vi "UI Chip Fitting.vi"(8 "error in":errorcluster) -> (0 "error out":errorcluster)   [LabVIEW 2019, in "Test.lvlib"]
uses:
  Test.lvlib
  Fluidic Process/SubVI/Fluidic Para.ctl
  <vilib>/Utility/file.llb/Read Delimited Spreadsheet (string).vi
  Controller/Controller.lvlib
  Queues/Queues.lvlib
  Fluidic Process/Fluidic Process.lvlib
  IO/sbRIO9623/sbRIO9623.lvlib
  Selection Valve/IDEX/IDEX.lvlib
panel:
  out "SW 2":bool
  out "SW 1":bool
  out "FW 2":bool
  out "FW 1":bool
  out "REA":bool
  out "V1":bool
  out "V2":bool
  out "BR1":bool
  out "BR2":bool
  out "BL1":bool
  out "BL2":bool
  in  "Air Tight":bool
  in  "Purge":bool
  in  "Flow Rate":bool
  in  "Chip Hold Pressure":bool
  in  "SW1/2":bool
  in  "FW1/2":bool
  in  "REA":bool
  in  "V1+BR1":bool
  in  "V2+BR2":bool
  in  "BR1":bool
  in  "BR2":bool
  in  "BL1":bool
  in  "BL2":bool
  in  "Stop Process":bool
  out "Remaining Time(s)":dbl
  out "Total Process":string
  out "Current Process":string
  out "Gauge":dbl(knob)=1.2869315802184793e-48 scale=0.0..100.0
  in  "Buffer Load R":bool
  in  "Buffer Load L":bool
  in  "Back":bool
  # "/"
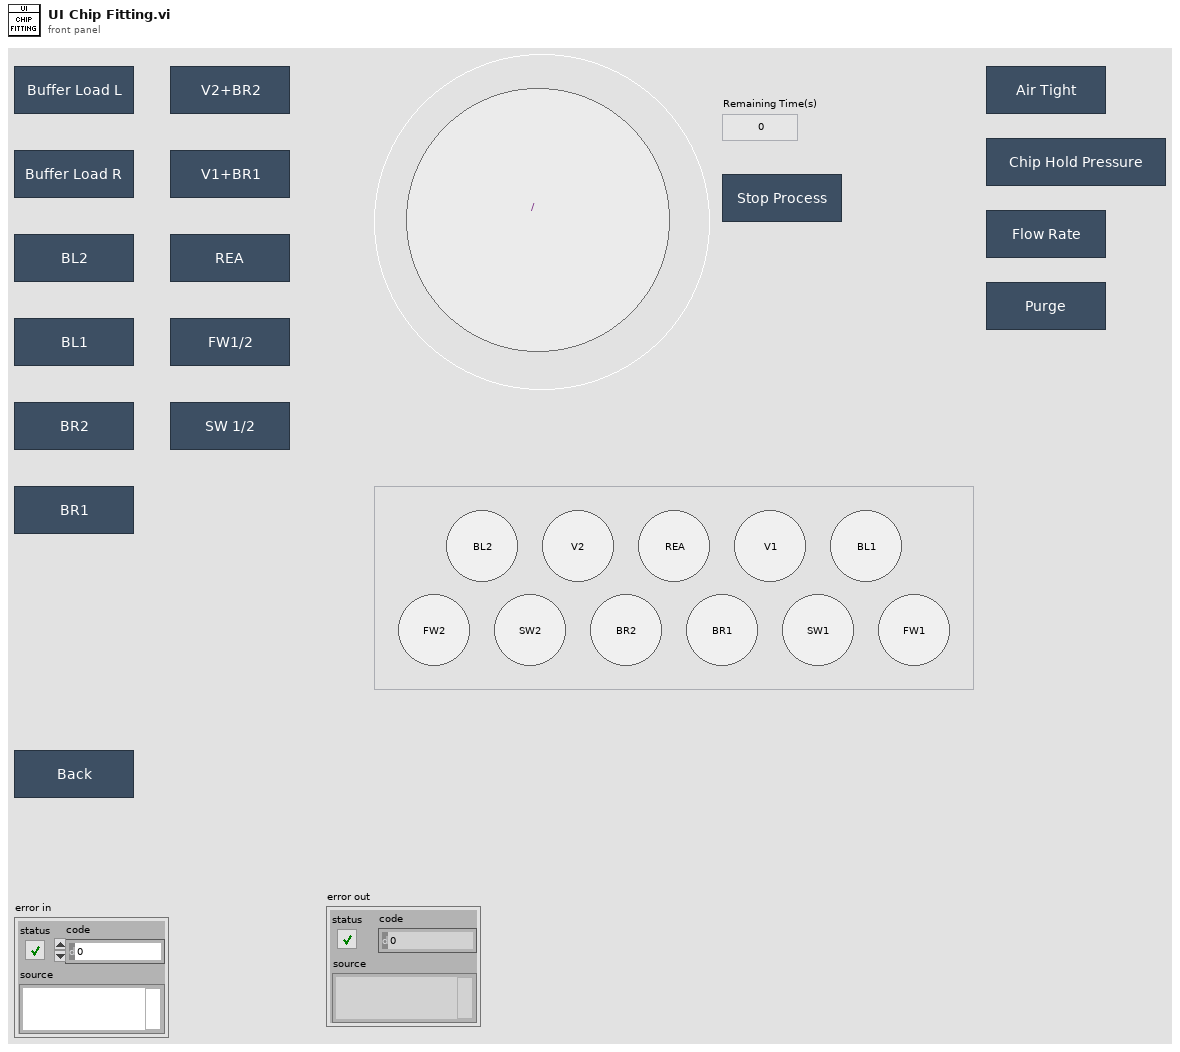
[diagram p1: front panel]
types:
  T1 = enum8{"Enabled", "Disabled", "Disabled and Grayed Out"}
  T2 = typedef "Fluidic Process.lvlib/Fluidic Para.ctl" = cluster{"Read Force Sensor":i32, "Read Regulator":i32, "Read Force Sensor?":bool, "Read Regulator?":bool, "Read Syringe Pump":i32, "Read Syringe Pump?":bool}
  T3 = enum16{"No Action", "Position 1", "Position 2", "Position 3", "Position 4", "Position 5", "Position 6"}
  T4 = typedef "Fluidic Process.lvlib/SEQ Data.ctl" = cluster{"Fluidic Process Done?":bool, "Current Process":i32, "Remaining Time":dbl, "Total Process":i32, "Air Sealing":bool, "Force Condition":bool}
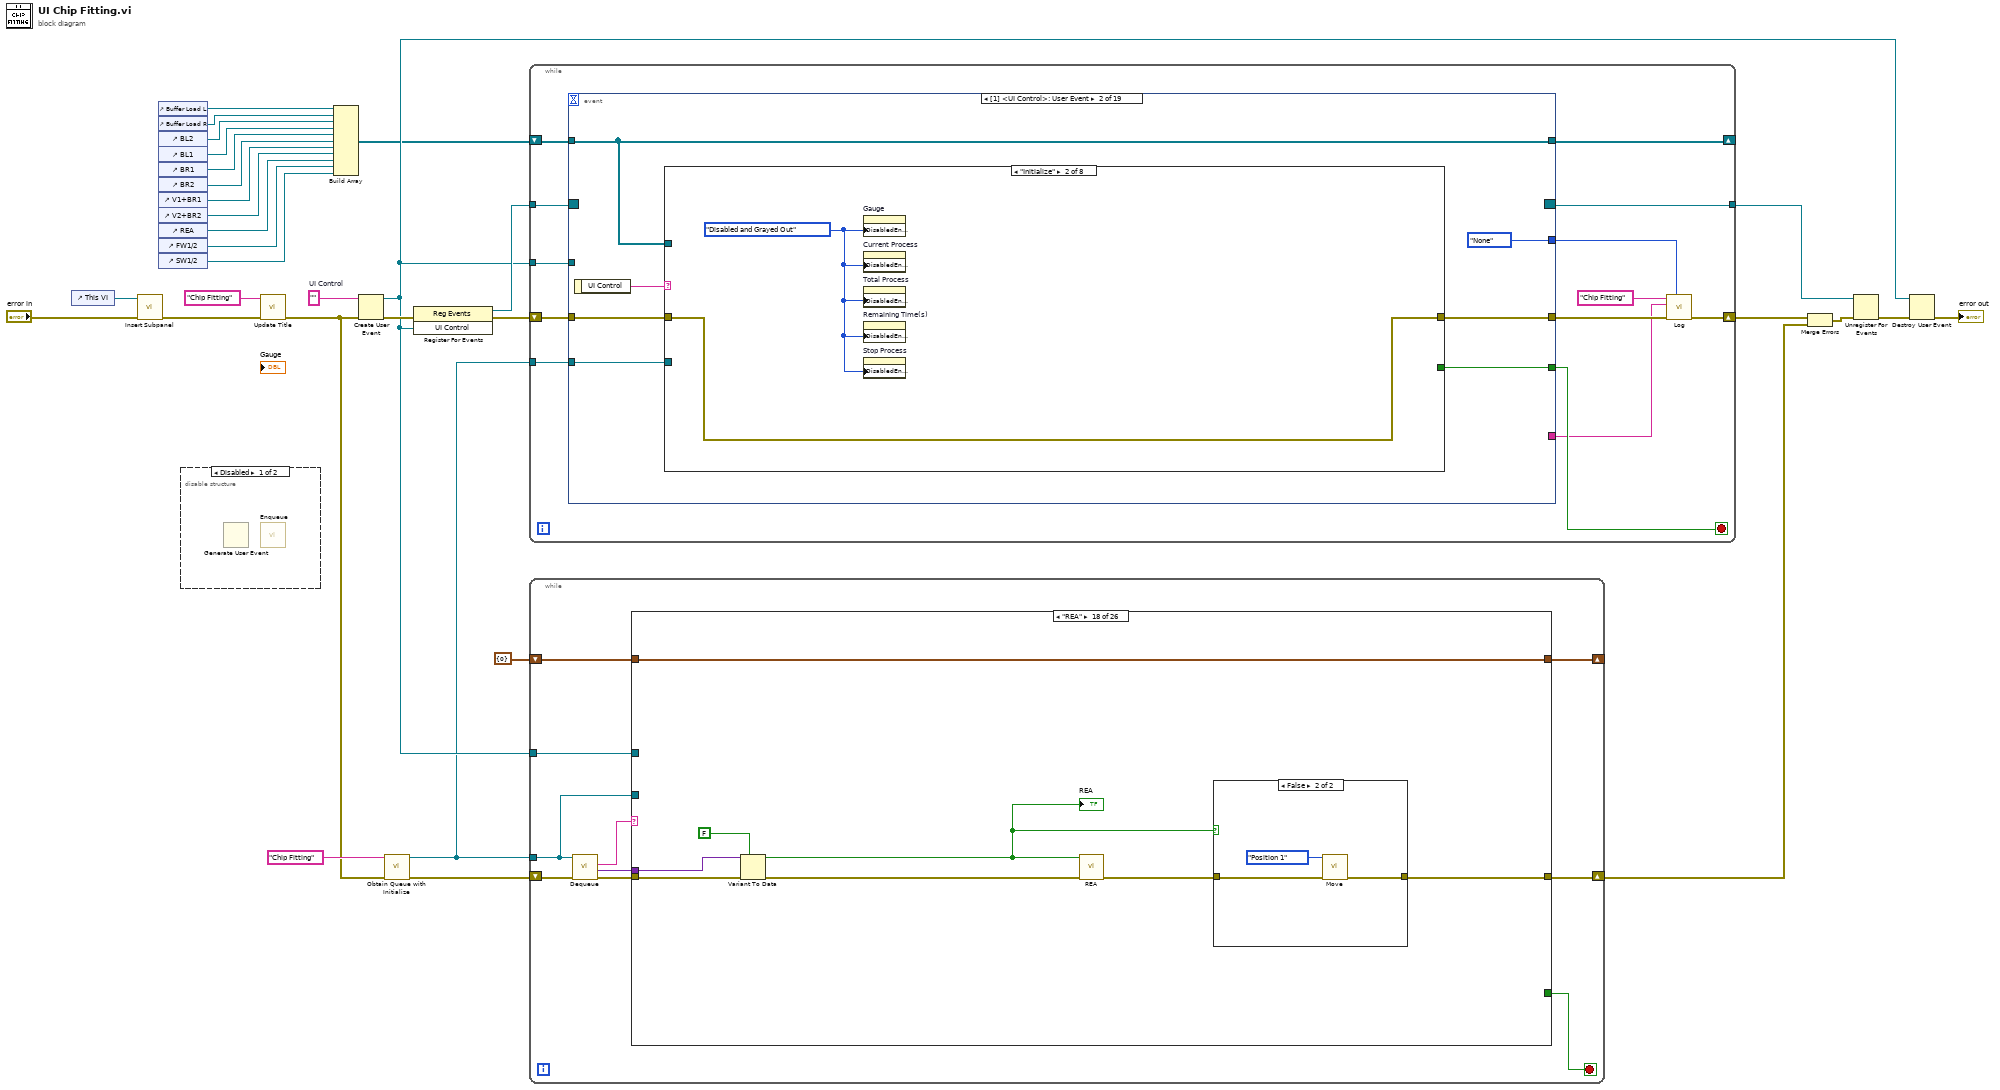
[diagram p0: block diagram]
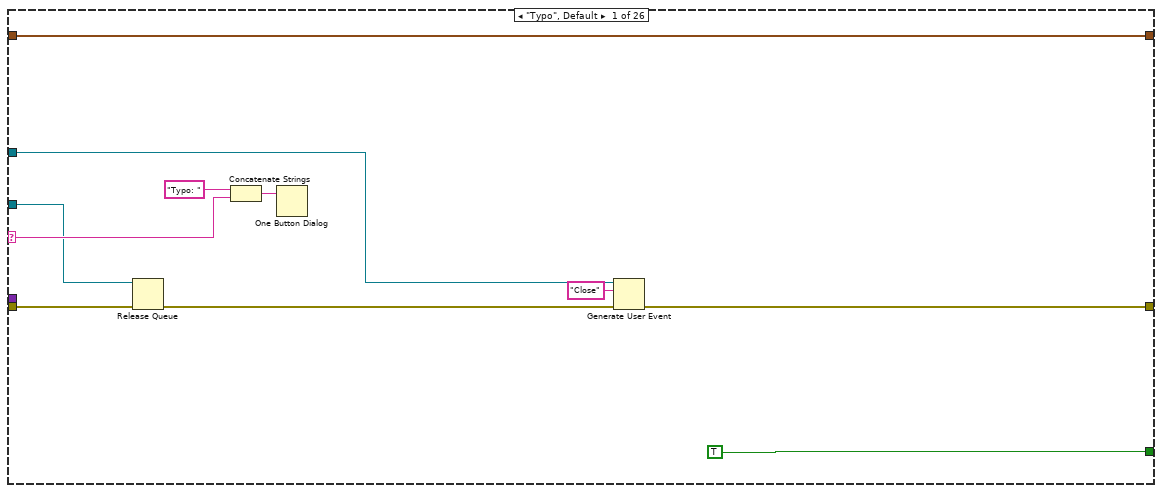
[diagram p3: hidden frame]
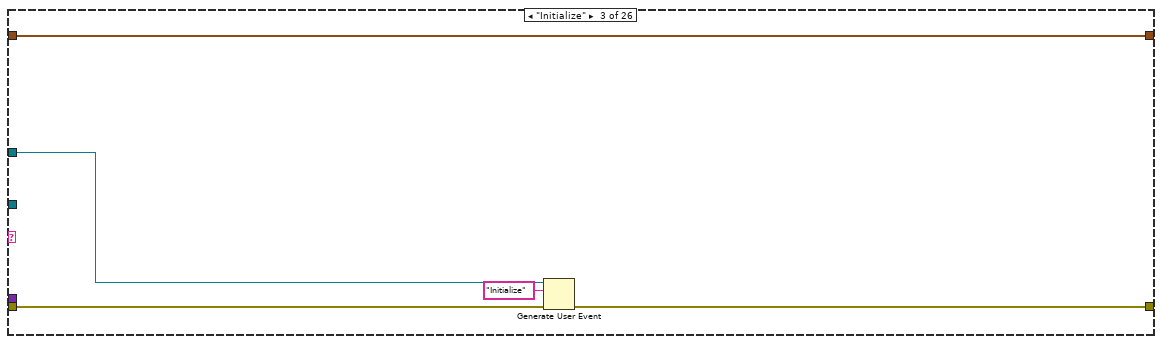
[diagram p5: hidden frame]
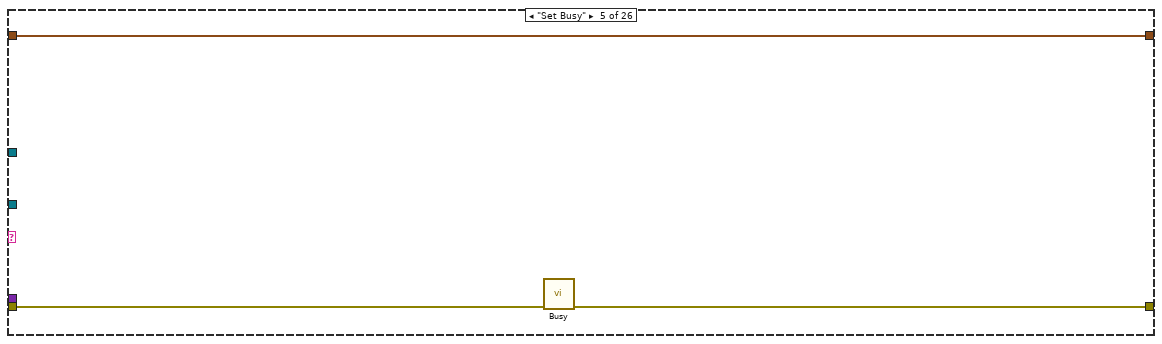
[diagram p7: hidden frame]
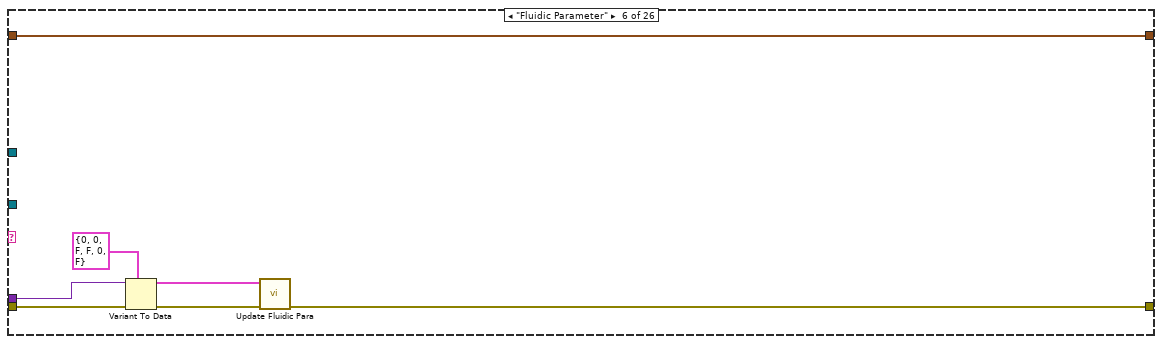
[diagram p8: hidden frame]
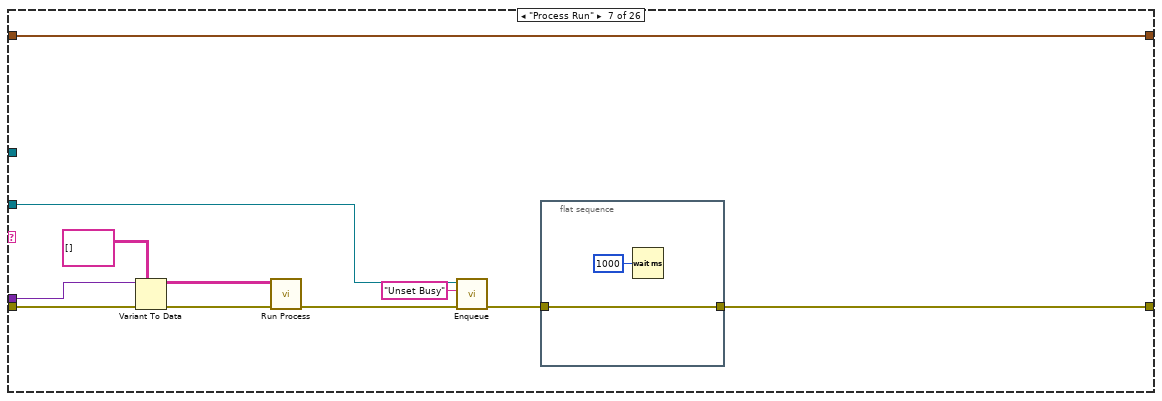
[diagram p9: hidden frame]
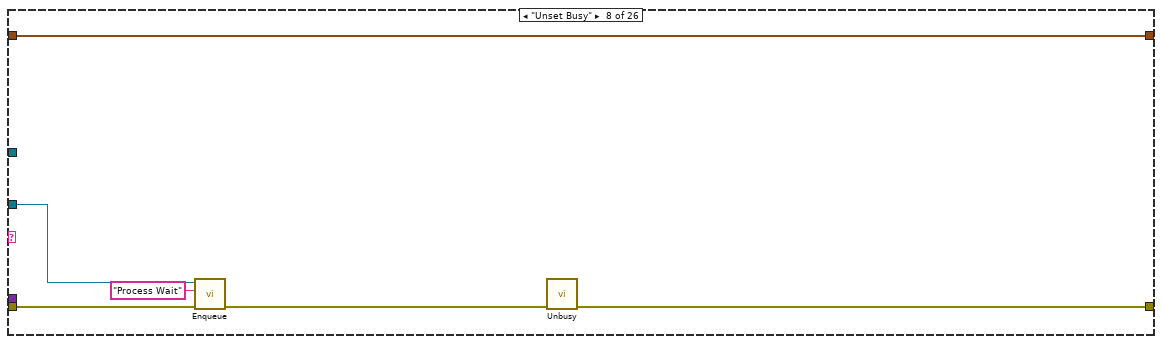
[diagram p10: hidden frame]
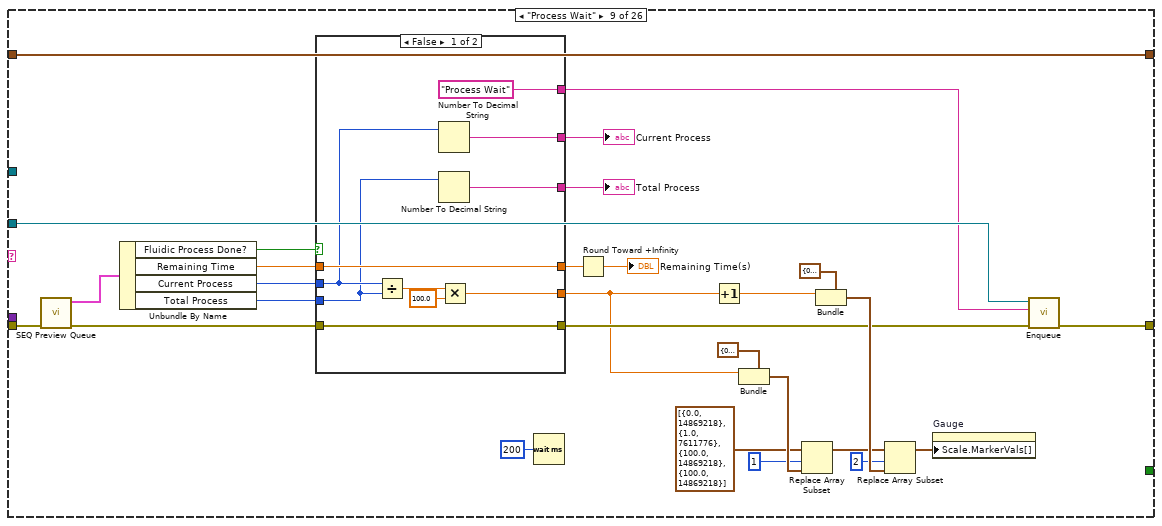
[diagram p11: hidden frame]
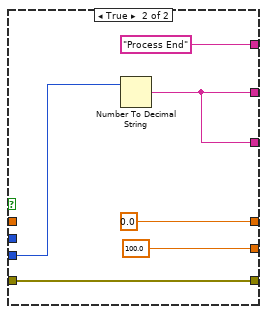
[diagram p12: hidden frame]
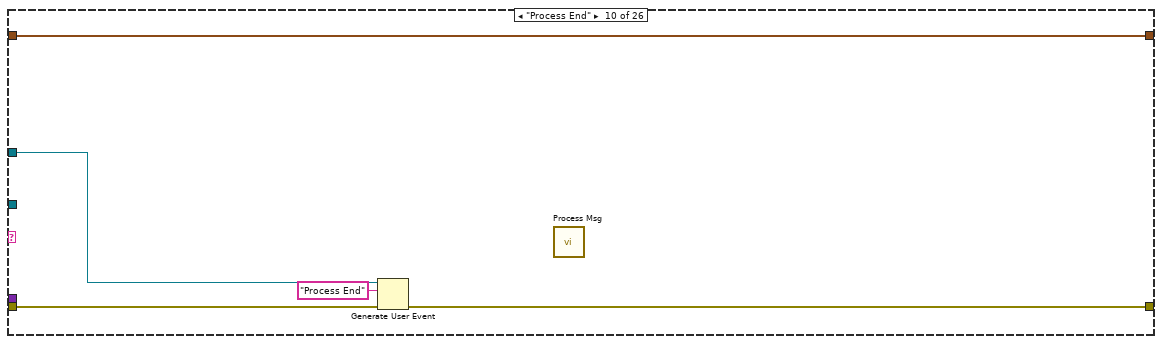
[diagram p13: hidden frame]
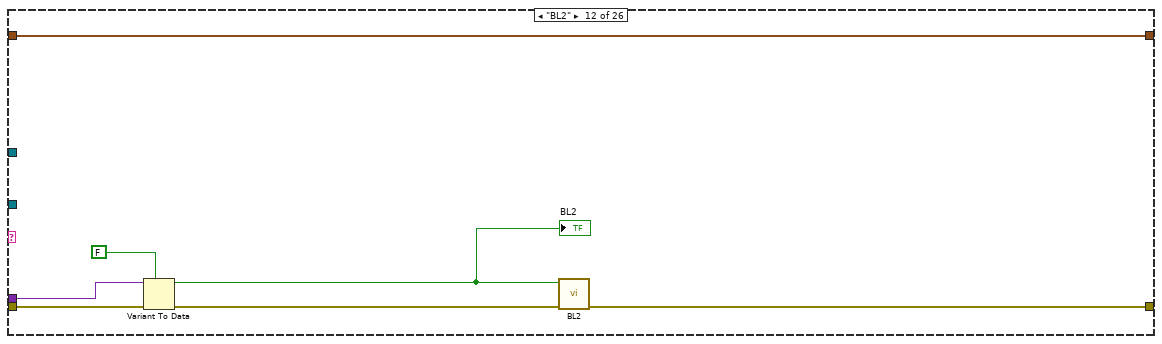
[diagram p15: hidden frame]
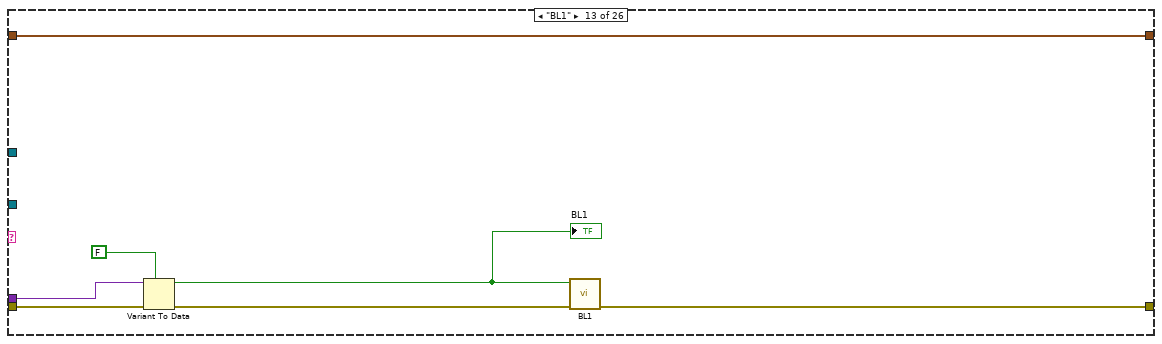
[diagram p16: hidden frame]
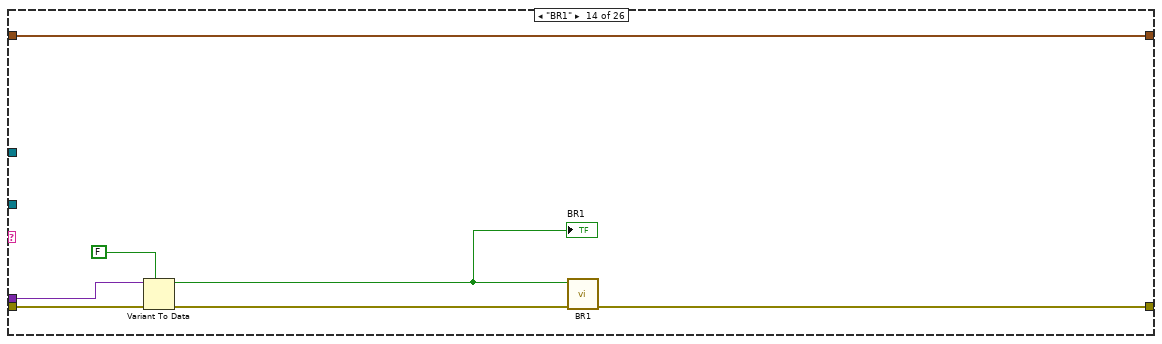
[diagram p17: hidden frame]
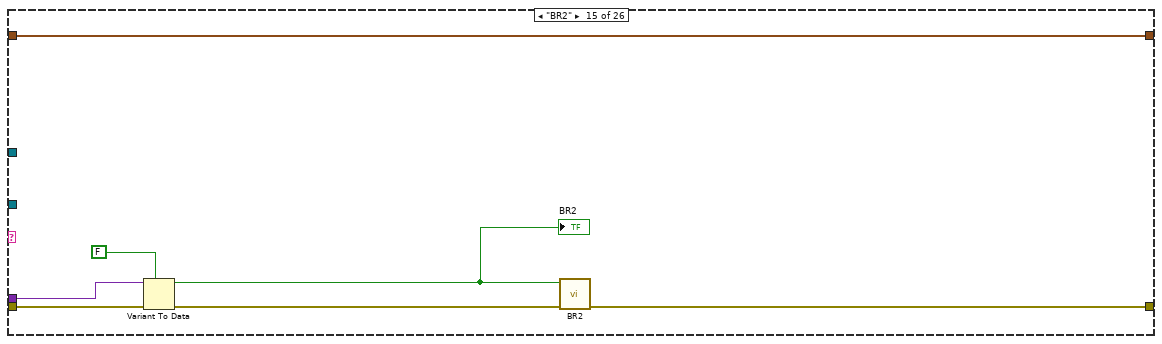
[diagram p18: hidden frame]
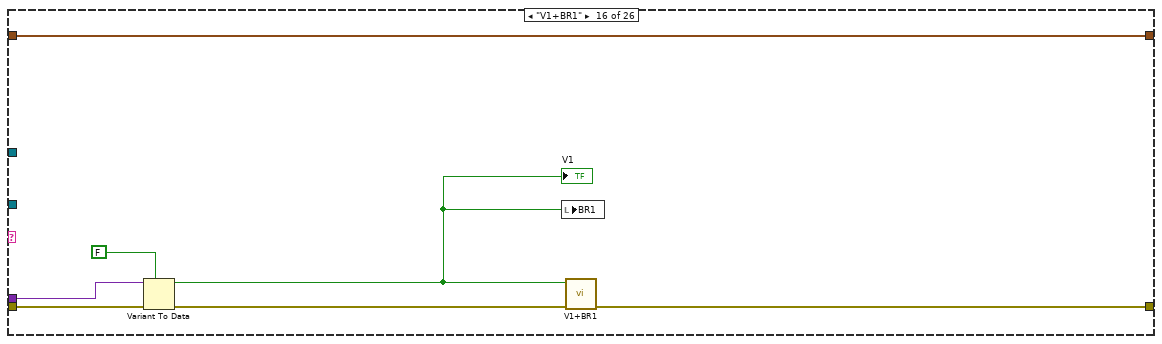
[diagram p19: hidden frame]
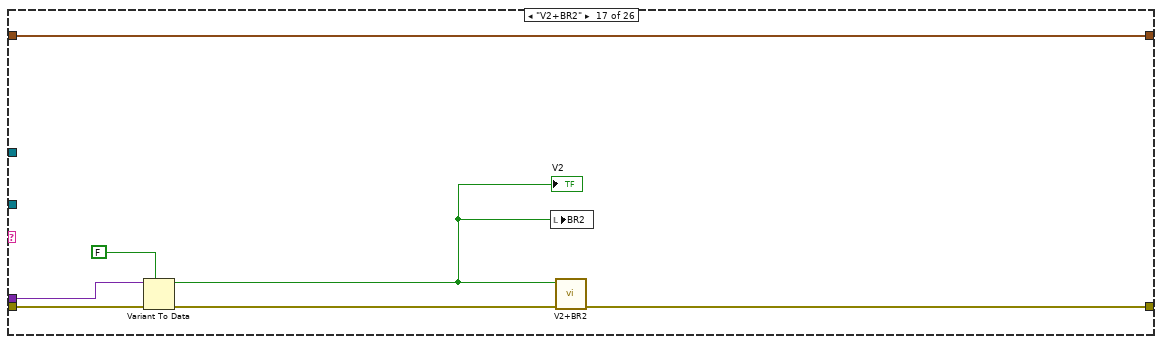
[diagram p20: hidden frame]
diagram:
  w22 = ""  # UI Control
  n1 = control-ref of="This VI"() -> (w21:refnum<vi>)
  n2 = call "Insert Subpanel.vi"("Error In"="error in", "VI Refnum"=w21) -> ("Error Out"=w15:errorcluster)  [unwired: 9 in]
  n3 = control-ref of="Buffer Load L"() -> (w12:refnum<vi>)
  n4 = control-ref of="Buffer Load R"() -> (w11:refnum<vi>)
  n5 = control-ref of="BL2"() -> (w10:refnum<vi>)
  n6 = control-ref of="BL1"() -> (w9:refnum<vi>)
  n7 = control-ref of="BR1"() -> (w8:refnum<vi>)
  n8 = control-ref of="BR2"() -> (w7:refnum<vi>)
  n9 = control-ref of="V1+BR1"() -> (w6:refnum<vi>)
  n10 = control-ref of="V2+BR2"() -> (w5:refnum<vi>)
  n11 = control-ref of="REA"() -> (w4:refnum<vi>)
  n12 = control-ref of="FW1/2"() -> (w3:refnum<vi>)
  n13 = control-ref of="SW1/2"() -> (w2:refnum<vi>)
  n14 = disable-structure shown="Disabled" {
    frame Disabled {
      n15 = Generate User Event() -> ()  [unwired: 4 in, 2 out]
      n16 = call "Enqueue.vi"() -> ()  [unwired: 10 in, 2 out]
    }
    frame Enabled {
    }
  }
  n17 = call "Update Title.vi"("Error In"=w15, "Title"="Chip Fitting") -> ("Error Out"=w14:errorcluster)  [unwired: 9 in]
  n18 = Build Array(w12, w11, w10, w9, w8, w7, w6, w5, w4, w3, w2) -> (w1:refnum<vi>[])
  n19 = Create User Event(user event datatype=w22, error in=w14) -> (user event=w20:refnum<user-event>, error out=w31:errorcluster)
  n20 = call "Obtain Queue with Initialize.vi"("Error In"=w14, "Queue Name"="Chip Fitting") -> ("Error Out"=w19:errorcluster, "Queue out"=w18:refnum<queue>)  [unwired: 8 in]
  n21 = register-events(error in=w31, w20) -> (reference out=w29:refnum<event-registration>, error out=w30:errorcluster)  [unwired: 1 in]
  n22 = while {
    tunnel: w29 -> [w43]
    tunnel: w18 -> [w42]
    shift-right: [w38] -> w27
    shift-left: w30 -> [w45]
    tunnel: [w41] -> w25
    tunnel: w20 -> [w40]
    shift-right: [w33] -> _
    shift-left: w1 -> [w34]
    stop <- w44 stop-if-true
    n23 = event shown="[1] <UI Control>: User Event" {
      selector: w43 -> [_ _ _ _ _ _ _ _ _ _ _ _ _ _ _ _ _ _ _]
      dyn-events: [_ _ _ _ _ _ _ _ _ _ _ _ _ _ _ _ _ _ _] -> w41
      timeout: _ -> [_ _ _ _ _ _ _ _ _ _ _ _ _ _ _ _ _ _ _]
      tunnel: w45 -> [w47 w54 w108 w138 w168 w198 w228 w236 w246 w256 w266 w276 w286 w296 w306 w316 w326 w332 w337]
      tunnel: [_ w50 _ _ _ _ _ _ _ _ _ _ _ _ _ _ _ _ TRUE] -> w44
      tunnel: w42 -> [_ w52 w119 w149 w179 w209 w226 w234 w244 w254 w264 w274 w284 w294 w304 w314 w324 _ w339]
      tunnel: [w47 w51 w115 w145 w175 w205 w227 w235 w245 w255 w265 w275 w285 w295 w305 w315 w325 w331 w340] -> w39
      tunnel: w40 -> [_ _ w106 w136 w166 w196 _ _ _ _ _ _ _ _ _ _ _ _ _]
      tunnel: [_ enum16{"None", "Write"}."None" ("Action") enum16{"None", "Write"}."Write" ("Action") enum16{"None", "Write"}."Write" ("Action") enum16{"None", "Write"}."Write" ("Action") enum16{"None", "Write"}."Write" ("Action") enum16{"None", "Write"}."Write" ("Action") enum16{"None", "Write"}."Write" ("Action") enum16{"None", "Write"}."Write" ("Action") enum16{"None", "Write"}."Write" ("Action") enum16{"None", "Write"}."Write" ("Action") enum16{"None", "Write"}."Write" ("Action") enum16{"None", "Write"}."Write" ("Action") enum16{"None", "Write"}."Write" ("Action") enum16{"None", "Write"}."Write" ("Action") enum16{"None", "Write"}."Write" ("Action") enum16{"None", "Write"}."Write" ("Action") enum16{"None", "Write"}."Write" ("Action") enum16{"None", "Write"}."Write" ("Action")] -> w36
      tunnel: [_ _ w103 w133 w163 w193 w222 w230 w238 w248 w258 w268 w278 w288 w298 w308 w318 w328 w335] -> w35
      tunnel: w34 -> [w46 w48 w101 w131 w161 w191 w221 w229 w237 w247 w257 w267 w277 w287 w297 w307 w317 w327 w333]
      tunnel: [w46 w48 w101 w131 w161 w191 w221 w229 w237 w247 w257 w267 w277 w287 w297 w307 w317 w327 w333] -> w33
      event Timeout {
        n24 = event-data() -> ()  [unwired: 1 in, 3 out]
      }
      event User Event {
        n25 = event-data() -> ("UI Control"=w53:string)  [unwired: 1 in]
        n26 = case shown="\"Initialize\"" w53 {
          selector: w53 -> [w57 _ _ _ _ _ _ _]
          tunnel: w54 -> [w62 w64 w69 w76 w83 w90 w96 w100]
          tunnel: w52 -> [w61 _ _ _ _ _ _ _]
          tunnel: [w56 w64 w69 w76 w83 w90 w96 w100] -> w51
          tunnel: [TRUE _ _ _ _ _ _ TRUE] -> w50
          tunnel: w48 -> [_ _ w65 w72 w79 w86 w93 _]
          frame "Typo", Default {
            n27 = Concatenate Strings("Typo: " ("string"), w57) -> (w58:string)
            n28 = One Button Dialog(message=w58) -> ()  [unwired: 1 in, 1 out]
            n29 = call "Enqueue.vi"("Error In"=w62, "State"="Close", "Queue in"=w61) -> ("Error Out"=w56:errorcluster)  [unwired: 7 in, 1 out]
          }
          frame "Initialize" {
            w63 = T1."Disabled and Grayed Out" ("Disabled")
            n30 = property on="Gauge" class="Knob (strict)"("DisabledEnum"=w63) -> ()  [unwired: 2 in, 2 out]
            n31 = property on="Current Process" class="Str"("DisabledEnum"=w63) -> ()  [unwired: 2 in, 2 out]
            n32 = property on="Total Process" class="Str"("DisabledEnum"=w63) -> ()  [unwired: 2 in, 2 out]
            n33 = property on="Remaining Time(s)" class="DigNum (strict)"("DisabledEnum"=w63) -> ()  [unwired: 2 in, 2 out]
            n34 = property on="Stop Process" class="Bool"("DisabledEnum"=w63) -> ()  [unwired: 2 in, 2 out]
          }
          frame "Chip Hold Pressure" {
            w68 = T1."Enabled" ("Disabled")
            w66 = T1."Disabled and Grayed Out" ("Disabled")
            n35 = for {
              tunnel: w65 -> [w71] mode=indexing
              n36 = property class="Bool"(reference=w71, "DisabledEnum"=T1."Disabled and Grayed Out" ("Disabled")) -> ()  [unwired: 1 in, 2 out]
            }
            n37 = property on="Gauge" class="Knob (strict)"("DisabledEnum"=w68) -> ()  [unwired: 2 in, 2 out]
            n38 = property on="Current Process" class="Str"("DisabledEnum"=w68) -> ()  [unwired: 2 in, 2 out]
            n39 = property on="Total Process" class="Str"("DisabledEnum"=w68) -> ()  [unwired: 2 in, 2 out]
            n40 = property on="Remaining Time(s)" class="DigNum (strict)"("DisabledEnum"=w68) -> ()  [unwired: 2 in, 2 out]
            n41 = property on="Stop Process" class="Bool"("DisabledEnum"=w68) -> ()  [unwired: 2 in, 2 out]
            n42 = property on="Chip Hold Pressure" class="Bool"("DisabledEnum"=T1."Enabled" ("Disabled")) -> ()  [unwired: 2 in, 2 out]
            n43 = property on="Flow Rate" class="Bool"("DisabledEnum"=w66) -> ()  [unwired: 2 in, 2 out]
            n44 = property on="Purge" class="Bool"("DisabledEnum"=w66) -> ()  [unwired: 2 in, 2 out]
            n45 = property on="Air Tight" class="Bool"("DisabledEnum"=w66) -> ()  [unwired: 2 in, 2 out]
            n46 = property on="Back" class="Bool"("DisabledEnum"=w66) -> ()  [unwired: 2 in, 2 out]
          }
          frame "Air Tight" {
            w75 = T1."Enabled" ("Disabled")
            w73 = T1."Disabled and Grayed Out" ("Disabled")
            n47 = for {
              tunnel: w72 -> [w78] mode=indexing
              n48 = property class="Bool"(reference=w78, "DisabledEnum"=T1."Disabled and Grayed Out" ("Disabled")) -> ()  [unwired: 1 in, 2 out]
            }
            n49 = property on="Gauge" class="Knob (strict)"("DisabledEnum"=w75) -> ()  [unwired: 2 in, 2 out]
            n50 = property on="Current Process" class="Str"("DisabledEnum"=w75) -> ()  [unwired: 2 in, 2 out]
            n51 = property on="Total Process" class="Str"("DisabledEnum"=w75) -> ()  [unwired: 2 in, 2 out]
            n52 = property on="Remaining Time(s)" class="DigNum (strict)"("DisabledEnum"=w75) -> ()  [unwired: 2 in, 2 out]
            n53 = property on="Stop Process" class="Bool"("DisabledEnum"=w75) -> ()  [unwired: 2 in, 2 out]
            n54 = property on="Chip Hold Pressure" class="Bool"("DisabledEnum"=w73) -> ()  [unwired: 2 in, 2 out]
            n55 = property on="Flow Rate" class="Bool"("DisabledEnum"=w73) -> ()  [unwired: 2 in, 2 out]
            n56 = property on="Purge" class="Bool"("DisabledEnum"=w73) -> ()  [unwired: 2 in, 2 out]
            n57 = property on="Air Tight" class="Bool"("DisabledEnum"=T1."Enabled" ("Disabled")) -> ()  [unwired: 2 in, 2 out]
            n58 = property on="Back" class="Bool"("DisabledEnum"=w73) -> ()  [unwired: 2 in, 2 out]
          }
          frame "Flow Rate" {
            w82 = T1."Enabled" ("Disabled")
            w80 = T1."Disabled and Grayed Out" ("Disabled")
            n59 = for {
              tunnel: w79 -> [w85] mode=indexing
              n60 = property class="Bool"(reference=w85, "DisabledEnum"=T1."Disabled and Grayed Out" ("Disabled")) -> ()  [unwired: 1 in, 2 out]
            }
            n61 = property on="Gauge" class="Knob (strict)"("DisabledEnum"=w82) -> ()  [unwired: 2 in, 2 out]
            n62 = property on="Current Process" class="Str"("DisabledEnum"=w82) -> ()  [unwired: 2 in, 2 out]
            n63 = property on="Total Process" class="Str"("DisabledEnum"=w82) -> ()  [unwired: 2 in, 2 out]
            n64 = property on="Remaining Time(s)" class="DigNum (strict)"("DisabledEnum"=w82) -> ()  [unwired: 2 in, 2 out]
            n65 = property on="Stop Process" class="Bool"("DisabledEnum"=w82) -> ()  [unwired: 2 in, 2 out]
            n66 = property on="Chip Hold Pressure" class="Bool"("DisabledEnum"=w80) -> ()  [unwired: 2 in, 2 out]
            n67 = property on="Flow Rate" class="Bool"("DisabledEnum"=T1."Enabled" ("Disabled")) -> ()  [unwired: 2 in, 2 out]
            n68 = property on="Purge" class="Bool"("DisabledEnum"=w80) -> ()  [unwired: 2 in, 2 out]
            n69 = property on="Air Tight" class="Bool"("DisabledEnum"=w80) -> ()  [unwired: 2 in, 2 out]
            n70 = property on="Back" class="Bool"("DisabledEnum"=w80) -> ()  [unwired: 2 in, 2 out]
          }
          frame "Purge" {
            w89 = T1."Enabled" ("Disabled")
            w87 = T1."Disabled and Grayed Out" ("Disabled")
            n71 = for {
              tunnel: w86 -> [w92] mode=indexing
              n72 = property class="Bool"(reference=w92, "DisabledEnum"=T1."Disabled and Grayed Out" ("Disabled")) -> ()  [unwired: 1 in, 2 out]
            }
            n73 = property on="Gauge" class="Knob (strict)"("DisabledEnum"=w89) -> ()  [unwired: 2 in, 2 out]
            n74 = property on="Current Process" class="Str"("DisabledEnum"=w89) -> ()  [unwired: 2 in, 2 out]
            n75 = property on="Total Process" class="Str"("DisabledEnum"=w89) -> ()  [unwired: 2 in, 2 out]
            n76 = property on="Remaining Time(s)" class="DigNum (strict)"("DisabledEnum"=w89) -> ()  [unwired: 2 in, 2 out]
            n77 = property on="Stop Process" class="Bool"("DisabledEnum"=w89) -> ()  [unwired: 2 in, 2 out]
            n78 = property on="Chip Hold Pressure" class="Bool"("DisabledEnum"=w87) -> ()  [unwired: 2 in, 2 out]
            n79 = property on="Flow Rate" class="Bool"("DisabledEnum"=w87) -> ()  [unwired: 2 in, 2 out]
            n80 = property on="Purge" class="Bool"("DisabledEnum"=T1."Enabled" ("Disabled")) -> ()  [unwired: 2 in, 2 out]
            n81 = property on="Air Tight" class="Bool"("DisabledEnum"=w87) -> ()  [unwired: 2 in, 2 out]
            n82 = property on="Back" class="Bool"("DisabledEnum"=w87) -> ()  [unwired: 2 in, 2 out]
          }
          frame "Process End" {
            w95 = T1."Disabled and Grayed Out" ("Disabled")
            w94 = T1."Enabled" ("Disabled")
            n83 = for {
              tunnel: w93 -> [w98] mode=indexing
              n84 = property class="Bool"(reference=w98, "DisabledEnum"=T1."Enabled" ("Disabled")) -> ()  [unwired: 1 in, 2 out]
            }
            n85 = property on="Gauge" class="Knob (strict)"("DisabledEnum"=w95) -> ()  [unwired: 2 in, 2 out]
            n86 = property on="Current Process" class="Str"("DisabledEnum"=w95) -> ()  [unwired: 2 in, 2 out]
            n87 = property on="Total Process" class="Str"("DisabledEnum"=w95) -> ()  [unwired: 2 in, 2 out]
            n88 = property on="Remaining Time(s)" class="DigNum (strict)"("DisabledEnum"=w95) -> ()  [unwired: 2 in, 2 out]
            n89 = property on="Stop Process" class="Bool"("DisabledEnum"=w95) -> ()  [unwired: 2 in, 2 out]
            n90 = property on="Chip Hold Pressure" class="Bool"("DisabledEnum"=w94) -> ()  [unwired: 2 in, 2 out]
            n91 = property on="Flow Rate" class="Bool"("DisabledEnum"=w94) -> ()  [unwired: 2 in, 2 out]
            n92 = property on="Purge" class="Bool"("DisabledEnum"=w94) -> ()  [unwired: 2 in, 2 out]
            n93 = property on="Air Tight" class="Bool"("DisabledEnum"=w94) -> ()  [unwired: 2 in, 2 out]
            n94 = property on="Back" class="Bool"("DisabledEnum"=w94) -> ()  [unwired: 2 in, 2 out]
          }
          frame "Close" {
          }
        }
      }
      event "Air Tight": Value Change {
        n95 = event-data() -> ("CtlRef"=w104:refnum<vi>)  [unwired: 1 in]
        n96 = property class="Bool"(reference=w104) -> ("Label.Text"=w103:string)  [unwired: 1 in, 2 out]
        n97 = Generate User Event(user event=w106, event data cluster="Air Tight" ("event data"), error in=w108) -> (error out=w107:errorcluster)  [unwired: 1 in, 1 out]
        n98 = disable-structure shown="RUN_TIME_ENGINE==False, Default" {
          disable-tunnel: [w120 w123] -> w117
          frame condition #0 (active) {
            n99 = call <vilib>:"Application Directory.vi"() -> ("Application Directory"=w122:path)
            n100 = Build Path(base path=w122, name or relative path="Fluidic Process\\File\\Air Tight.txt") -> (appended path=w120:path)
          }
          frame condition #1 {
            n101 = call <vilib>:"Application Directory.vi"() -> ("Application Directory"=w125:path)
            n102 = Build Path(base path=w125, name or relative path="data\\File\\Air Tight.txt") -> (appended path=w123:path)
          }
        }
        n103 = call-poly <vilib>:"Read Delimited Spreadsheet.vi"("file path (dialog if empty)"=w117, "error in (no error)"=w107) -> ("all rows"=w116:string[][], "error out"=w118:errorcluster)  [unwired: 8 in, 4 out]
        n104 = To Variant(anything=T2 {"Read Force Sensor"=0, "Read Regulator"=2, "Read Force Sensor?"=FALSE, "Read Regulator?"=TRUE, "Read Syringe Pump"=0, "Read Syringe Pump?"=FALSE} ("Cluster")) -> (Variant=w111:variant)
        n105 = To Variant(anything=w116) -> (Variant=w113:variant)
        n106 = Build Array(variant, w111, w113) -> (w110:variant[])
        n107 = for {
          tunnel: w119 -> [w130]
          shift-right: [w128] -> w115
          shift-left: w118 -> [w129]
          tunnel: string[] ["Set Busy", "Fluidic Parameter", "Process Run"] -> [w127] mode=indexing
          tunnel: w110 -> [w126] mode=indexing
          n108 = call "Enqueue.vi"("Error In"=w129, "Data"=w126, "State"=w127, "Queue in"=w130) -> ("Error Out"=w128:errorcluster)  [unwired: 6 in, 1 out]
        }
      }
      event "Chip Hold Pressure": Value Change {
        n109 = event-data() -> ("CtlRef"=w134:refnum<vi>)  [unwired: 1 in]
        n110 = property class="Bool"(reference=w134) -> ("Label.Text"=w133:string)  [unwired: 1 in, 2 out]
        n111 = Generate User Event(user event=w136, event data cluster="Chip Hold Pressure" ("event data"), error in=w138) -> (error out=w137:errorcluster)  [unwired: 1 in, 1 out]
        n112 = disable-structure shown="RUN_TIME_ENGINE==False, Default" {
          disable-tunnel: [w150 w153] -> w147
          frame condition #0 (active) {
            n113 = call <vilib>:"Application Directory.vi"() -> ("Application Directory"=w152:path)
            n114 = Build Path(base path=w152, name or relative path="Fluidic Process\\File\\Chip Hold Pressure.txt") -> (appended path=w150:path)
          }
          frame condition #1 {
            n115 = call <vilib>:"Application Directory.vi"() -> ("Application Directory"=w155:path)
            n116 = Build Path(base path=w155, name or relative path="data\\File\\Chip Hold Pressure.txt") -> (appended path=w153:path)
          }
        }
        n117 = call-poly <vilib>:"Read Delimited Spreadsheet.vi"("file path (dialog if empty)"=w147, "error in (no error)"=w137) -> ("all rows"=w146:string[][], "error out"=w148:errorcluster)  [unwired: 8 in, 4 out]
        n118 = To Variant(anything=T2 {"Read Force Sensor"=0, "Read Regulator"=0, "Read Force Sensor?"=FALSE, "Read Regulator?"=FALSE, "Read Syringe Pump"=0, "Read Syringe Pump?"=FALSE} ("Cluster")) -> (Variant=w141:variant)
        n119 = To Variant(anything=w146) -> (Variant=w143:variant)
        n120 = Build Array(variant, w141, w143) -> (w140:variant[])
        n121 = for {
          tunnel: w149 -> [w160]
          shift-right: [w158] -> w145
          shift-left: w148 -> [w159]
          tunnel: string[] ["Set Busy", "Fluidic Parameter", "Process Run"] -> [w157] mode=indexing
          tunnel: w140 -> [w156] mode=indexing
          n122 = call "Enqueue.vi"("Error In"=w159, "Data"=w156, "State"=w157, "Queue in"=w160) -> ("Error Out"=w158:errorcluster)  [unwired: 6 in, 1 out]
        }
      }
      event "Flow Rate": Value Change {
        n123 = event-data() -> ("CtlRef"=w164:refnum<vi>)  [unwired: 1 in]
        n124 = property class="Bool"(reference=w164) -> ("Label.Text"=w163:string)  [unwired: 1 in, 2 out]
        n125 = Generate User Event(user event=w166, event data cluster="Flow Rate" ("event data"), error in=w168) -> (error out=w167:errorcluster)  [unwired: 1 in, 1 out]
        n126 = disable-structure shown="RUN_TIME_ENGINE==False, Default" {
          disable-tunnel: [w180 w183] -> w177
          frame condition #0 (active) {
            n127 = call <vilib>:"Application Directory.vi"() -> ("Application Directory"=w182:path)
            n128 = Build Path(base path=w182, name or relative path="Fluidic Process\\File\\Flow Rate.txt") -> (appended path=w180:path)
          }
          frame condition #1 {
            n129 = call <vilib>:"Application Directory.vi"() -> ("Application Directory"=w185:path)
            n130 = Build Path(base path=w185, name or relative path="data\\File\\Flow Rate.txt") -> (appended path=w183:path)
          }
        }
        n131 = call-poly <vilib>:"Read Delimited Spreadsheet.vi"("file path (dialog if empty)"=w177, "error in (no error)"=w167) -> ("all rows"=w176:string[][], "error out"=w178:errorcluster)  [unwired: 8 in, 4 out]
        n132 = To Variant(anything=T2 {"Read Force Sensor"=0, "Read Regulator"=0, "Read Force Sensor?"=FALSE, "Read Regulator?"=FALSE, "Read Syringe Pump"=0, "Read Syringe Pump?"=FALSE} ("Cluster")) -> (Variant=w171:variant)
        n133 = To Variant(anything=w176) -> (Variant=w173:variant)
        n134 = Build Array(variant, w171, w173) -> (w170:variant[])
        n135 = for {
          tunnel: w179 -> [w190]
          shift-right: [w188] -> w175
          shift-left: w178 -> [w189]
          tunnel: string[] ["Set Busy", "Fluidic Parameter", "Process Run"] -> [w187] mode=indexing
          tunnel: w170 -> [w186] mode=indexing
          n136 = call "Enqueue.vi"("Error In"=w189, "Data"=w186, "State"=w187, "Queue in"=w190) -> ("Error Out"=w188:errorcluster)  [unwired: 6 in, 1 out]
        }
      }
      event "Purge": Value Change {
        n137 = event-data() -> ("CtlRef"=w194:refnum<vi>)  [unwired: 1 in]
        n138 = property class="Bool"(reference=w194) -> ("Label.Text"=w193:string)  [unwired: 1 in, 2 out]
        n139 = Generate User Event(user event=w196, event data cluster="Purge" ("event data"), error in=w198) -> (error out=w197:errorcluster)  [unwired: 1 in, 1 out]
        n140 = disable-structure shown="RUN_TIME_ENGINE==False, Default" {
          disable-tunnel: [w210 w213] -> w207
          frame condition #0 (active) {
            n141 = call <vilib>:"Application Directory.vi"() -> ("Application Directory"=w212:path)
            n142 = Build Path(base path=w212, name or relative path="Fluidic Process\\File\\Purge.txt") -> (appended path=w210:path)
          }
          frame condition #1 {
            n143 = call <vilib>:"Application Directory.vi"() -> ("Application Directory"=w215:path)
            n144 = Build Path(base path=w215, name or relative path="data\\File\\Purge.txt") -> (appended path=w213:path)
          }
        }
        n145 = call-poly <vilib>:"Read Delimited Spreadsheet.vi"("file path (dialog if empty)"=w207, "error in (no error)"=w197) -> ("all rows"=w206:string[][], "error out"=w208:errorcluster)  [unwired: 8 in, 4 out]
        n146 = To Variant(anything=T2 {"Read Force Sensor"=5, "Read Regulator"=0, "Read Force Sensor?"=TRUE, "Read Regulator?"=FALSE, "Read Syringe Pump"=6, "Read Syringe Pump?"=TRUE} ("Cluster")) -> (Variant=w201:variant)
        n147 = To Variant(anything=w206) -> (Variant=w203:variant)
        n148 = Build Array(variant, w201, w203) -> (w200:variant[])
        n149 = for {
          tunnel: w209 -> [w220]
          shift-right: [w218] -> w205
          shift-left: w208 -> [w219]
          tunnel: string[] ["Set Busy", "Fluidic Parameter", "Process Run"] -> [w217] mode=indexing
          tunnel: w200 -> [w216] mode=indexing
          n150 = call "Enqueue.vi"("Error In"=w219, "Data"=w216, "State"=w217, "Queue in"=w220) -> ("Error Out"=w218:errorcluster)  [unwired: 6 in, 1 out]
        }
      }
      event "Buffer Load L": Value Change {
        n151 = event-data() -> ("CtlRef"=w223:refnum<vi>)  [unwired: 1 in]
        n152 = property class="Bool"(reference=w223) -> ("Label.Text"=w222:string)  [unwired: 1 in, 2 out]
        n153 = call "Enqueue.vi"("Error In"=w228, "State"="Buffer Load L", "Queue in"=w226) -> ("Error Out"=w227:errorcluster)  [unwired: 7 in, 1 out]
      }
      event "Buffer Load R": Value Change {
        n154 = event-data() -> ("CtlRef"=w231:refnum<vi>)  [unwired: 1 in]
        n155 = property class="Bool"(reference=w231) -> ("Label.Text"=w230:string)  [unwired: 1 in, 2 out]
        n156 = call "Enqueue.vi"("Error In"=w236, "State"="Buffer Load R", "Queue in"=w234) -> ("Error Out"=w235:errorcluster)  [unwired: 7 in, 1 out]
      }
      event "BL2": Value Change {
        n157 = event-data() -> ("NewVal"=w243:bool, "CtlRef"=w239:refnum<vi>)  [unwired: 1 in]
        n158 = property class="Bool (strict)"(reference=w239) -> ("Label.Text"=w238:string)  [unwired: 1 in, 2 out]
        n159 = To Variant(anything=w243) -> (Variant=w242:variant)
        n160 = call "Enqueue.vi"("Error In"=w246, "Data"=w242, "State"="BL2", "Queue in"=w244) -> ("Error Out"=w245:errorcluster)  [unwired: 6 in, 1 out]
      }
      event "BL1": Value Change {
        n161 = event-data() -> ("NewVal"=w252:bool, "CtlRef"=w249:refnum<vi>)  [unwired: 1 in]
        n162 = property class="Bool (strict)"(reference=w249) -> ("Label.Text"=w248:string)  [unwired: 1 in, 2 out]
        n163 = To Variant(anything=w252) -> (Variant=w251:variant)
        n164 = call "Enqueue.vi"("Error In"=w256, "Data"=w251, "State"="BL1", "Queue in"=w254) -> ("Error Out"=w255:errorcluster)  [unwired: 6 in, 1 out]
      }
      event "BR1": Value Change {
        n165 = event-data() -> ("NewVal"=w262:bool, "CtlRef"=w259:refnum<vi>)  [unwired: 1 in]
        n166 = property class="Bool (strict)"(reference=w259) -> ("Label.Text"=w258:string)  [unwired: 1 in, 2 out]
        n167 = To Variant(anything=w262) -> (Variant=w261:variant)
        n168 = call "Enqueue.vi"("Error In"=w266, "Data"=w261, "State"="BR1", "Queue in"=w264) -> ("Error Out"=w265:errorcluster)  [unwired: 6 in, 1 out]
      }
      event "BR2": Value Change {
        n169 = event-data() -> ("NewVal"=w272:bool, "CtlRef"=w269:refnum<vi>)  [unwired: 1 in]
        n170 = property class="Bool (strict)"(reference=w269) -> ("Label.Text"=w268:string)  [unwired: 1 in, 2 out]
        n171 = To Variant(anything=w272) -> (Variant=w271:variant)
        n172 = call "Enqueue.vi"("Error In"=w276, "Data"=w271, "State"="BR2", "Queue in"=w274) -> ("Error Out"=w275:errorcluster)  [unwired: 6 in, 1 out]
      }
      event "V1+BR1": Value Change {
        n173 = event-data() -> ("NewVal"=w282:bool, "CtlRef"=w279:refnum<vi>)  [unwired: 1 in]
        n174 = property class="Bool (strict)"(reference=w279) -> ("Label.Text"=w278:string)  [unwired: 1 in, 2 out]
        n175 = To Variant(anything=w282) -> (Variant=w281:variant)
        n176 = call "Enqueue.vi"("Error In"=w286, "Data"=w281, "State"="V1+BR1", "Queue in"=w284) -> ("Error Out"=w285:errorcluster)  [unwired: 6 in, 1 out]
      }
      event "V2+BR2": Value Change {
        n177 = event-data() -> ("NewVal"=w292:bool, "CtlRef"=w289:refnum<vi>)  [unwired: 1 in]
        n178 = property class="Bool (strict)"(reference=w289) -> ("Label.Text"=w288:string)  [unwired: 1 in, 2 out]
        n179 = To Variant(anything=w292) -> (Variant=w291:variant)
        n180 = call "Enqueue.vi"("Error In"=w296, "Data"=w291, "State"="V2+BR2", "Queue in"=w294) -> ("Error Out"=w295:errorcluster)  [unwired: 6 in, 1 out]
      }
      event "REA": Value Change {
        n181 = event-data() -> ("NewVal"=w302:bool, "CtlRef"=w299:refnum<vi>)  [unwired: 1 in]
        n182 = property class="Bool (strict)"(reference=w299) -> ("Label.Text"=w298:string)  [unwired: 1 in, 2 out]
        n183 = To Variant(anything=w302) -> (Variant=w301:variant)
        n184 = call "Enqueue.vi"("Error In"=w306, "Data"=w301, "State"="REA", "Queue in"=w304) -> ("Error Out"=w305:errorcluster)  [unwired: 6 in, 1 out]
      }
      event "FW1/2": Value Change {
        n185 = event-data() -> ("NewVal"=w312:bool, "CtlRef"=w309:refnum<vi>)  [unwired: 1 in]
        n186 = property class="Bool (strict)"(reference=w309) -> ("Label.Text"=w308:string)  [unwired: 1 in, 2 out]
        n187 = To Variant(anything=w312) -> (Variant=w311:variant)
        n188 = call "Enqueue.vi"("Error In"=w316, "Data"=w311, "State"="FW1/2", "Queue in"=w314) -> ("Error Out"=w315:errorcluster)  [unwired: 6 in, 1 out]
      }
      event "SW1/2": Value Change {
        n189 = event-data() -> ("NewVal"=w322:bool, "CtlRef"=w319:refnum<vi>)  [unwired: 1 in]
        n190 = property class="Bool (strict)"(reference=w319) -> ("Label.Text"=w318:string)  [unwired: 1 in, 2 out]
        n191 = To Variant(anything=w322) -> (Variant=w321:variant)
        n192 = call "Enqueue.vi"("Error In"=w326, "Data"=w321, "State"="SW1/2", "Queue in"=w324) -> ("Error Out"=w325:errorcluster)  [unwired: 6 in, 1 out]
      }
      event "Stop Process": Value Change {
        n193 = event-data() -> ("CtlRef"=w329:refnum<vi>)  [unwired: 1 in]
        n194 = property class="Bool"(reference=w329) -> ("Label.Text"=w328:string)  [unwired: 1 in, 2 out]
        n195 = call "Stop Process.vi"("Error In"=w332) -> ("Error Out"=w331:errorcluster)  [unwired: 10 in]
      }
      event "Back": Value Change {
        n196 = event-data() -> ("CtlRef"=w336:refnum<vi>)  [unwired: 1 in]
        n197 = property class="Bool"(reference=w336) -> ("Label.Text"=w335:string)  [unwired: 1 in, 2 out]
        n198 = call "Enqueue.vi"("Error In"=w337, "State"="Close", "Queue in"=w339) -> ("Error Out"=w340:errorcluster)  [unwired: 7 in, 1 out]
      }
    }
    n199 = call "Log.vi"("Action"=w36, "error in"=w39, "State"=w35, "Page Name"="Chip Fitting") -> ("error out"=w38:errorcluster)  [unwired: 7 in]
  }
  n200 = while {
    tunnel: w18 -> [w348]
    shift-right: [w346] -> w26
    shift-left: w19 -> [w351]
    tunnel: w20 -> [w345]
    shift-right: [w342] -> _
    shift-left: cluster{"Tick Count":u32} {"Tick Count"=0} -> [w343]
    stop <- w344 stop-if-true
    n201 = call "Dequeue.vi"("Error In"=w351, "Queue in"=w348) -> ("Error Out"=w347:errorcluster, "Data"=w349:variant, "State"=w350:string)  [unwired: 6 in, 1 out]
    n202 = case shown="\"REA\"" w350 {
      selector: w350 -> [w360 _ _ _ _ _ _ _ _ _ _ _ _ _ _ _ _ _ _ _ _ _ _ _ _ _]
      tunnel: w349 -> [_ _ _ _ _ w380 w391 _ _ _ _ w456 w463 w470 w477 w484 w491 w499 w512 w519 _ _ _ _ _ _]
      tunnel: w348 -> [w353 _ _ _ _ _ w386 w399 w407 _ _ _ _ _ _ _ _ _ _ _ w528 w533 w558 w561 _ w582]
      tunnel: w347 -> [w355 w364 w369 w371 w373 w381 w392 w400 w428 w449 w451 w457 w464 w471 w478 w485 w492 w500 w513 w520 w523 w535 w551 w563 w578 w584]
      tunnel: [TRUE _ _ _ _ _ _ _ _ _ _ _ _ _ _ _ _ _ _ _ _ _ _ _ _ TRUE] -> w344
      tunnel: [w358 w364 w368 w371 w372 w376 w383 w395 w412 w448 w451 w453 w460 w467 w474 w481 w488 w495 w509 w516 w526 w534 w553 w562 w578 w583] -> w346
      tunnel: w345 -> [w357 _ w367 _ _ _ _ _ _ w447 _ _ _ _ _ _ _ _ _ _ _ _ _ _ _ _]
      tunnel: w343 -> [w352 w363 w365 w370 w374 w375 w382 w397 w403 w445 w450 w458 w465 w472 w479 w486 w493 w501 w514 w521 w531 w541 w559 w569 w579 w580]
      tunnel: [w352 w363 w365 w370 w374 w375 w382 w397 w403 w445 w450 w458 w465 w472 w479 w486 w493 w501 w514 w521 w525 w541 w556 w569 w579 w580] -> w342
      frame "Typo", Default {
        n203 = Release Queue(queue=w353, error in (no error)=w355) -> (error out=w354:errorcluster)  [unwired: 1 in, 2 out]
        n204 = Concatenate Strings("Typo: " ("string"), w360) -> (w362:string)
        n205 = One Button Dialog(message=w362) -> ()  [unwired: 1 in, 1 out]
        n206 = Generate User Event(user event=w357, event data cluster="Close" ("event data"), error in=w354) -> (error out=w358:errorcluster)  [unwired: 1 in, 1 out]
      }
      frame "------Initialize------" {
      }
      frame "Initialize" {
        n207 = Generate User Event(user event=w367, event data cluster="Initialize" ("event data"), error in=w369) -> (error out=w368:errorcluster)  [unwired: 1 in, 1 out]
      }
      frame "------Process------" {
      }
      frame "Set Busy" {
        n208 = call "Busy.vi"("Error In"=w373) -> ("Error Out"=w372:errorcluster)  [unwired: 10 in]
      }
      frame "Fluidic Parameter" {
        n209 = Variant To Data(error in=w381, type=T2 {"Read Force Sensor"=0, "Read Regulator"=0, "Read Force Sensor?"=FALSE, "Read Regulator?"=FALSE, "Read Syringe Pump"=0, "Read Syringe Pump?"=FALSE} ("Cluster"), Variant=w380) -> (data=w377:T2, error out=w378:errorcluster)
        n210 = call "Update Fluidic Para.vi"("Error In"=w378, "Fluidic Para"=w377) -> ("Error Out"=w376:errorcluster)  [unwired: 9 in]
      }
      frame "Process Run" {
        n211 = Variant To Data(error in=w392, type=string[][] [] ("all rows"), Variant=w391) -> (data=w388:string[][], error out=w389:errorcluster)
        n212 = call "Run Process.vi"("Error In"=w389, "Fluidic Process in"=w388) -> ("Error Out"=w387:errorcluster)  [unwired: 9 in]
        n213 = call "Enqueue.vi"("Error In"=w387, "State"="Unset Busy", "Queue in"=w386) -> ("Error Out"=w384:errorcluster)  [unwired: 7 in, 1 out]
        n214 = flat-sequence {
          tunnel: w384 -> [w394]
          tunnel: [w394] -> w383
          frame #0 {
            n215 = Wait (ms)(milliseconds to wait=u32 1000) -> ()  [unwired: 1 out]
          }
        }
      }
      frame "Unset Busy" {
        n216 = call "Enqueue.vi"("Error In"=w400, "State"="Process Wait", "Queue in"=w399) -> ("Error Out"=w396:errorcluster)  [unwired: 7 in, 1 out]
        n217 = call "Unbusy.vi"("Error In"=w396) -> ("Error Out"=w395:errorcluster)  [unwired: 10 in]
      }
      frame "Process Wait" {
        n218 = call "SEQ Preview Queue.vi"("error in"=w428) -> ("error out"=w425:errorcluster, "SEQ Data"=w427:T4)  [unwired: 9 in]
        n219 = Unbundle By Name(w427) -> ("Fluidic Process Done?"=w426:bool, "Remaining Time"=w411:dbl, "Current Process"=w410:i32, "Total Process"=w409:i32)
        n220 = case shown="False" w426 {
          tunnel: w425 -> [w436 w444]
          tunnel: [w436 w444] -> w413
          tunnel: w411 -> [w435 _]
          tunnel: w410 -> [w433 _]
          tunnel: w409 -> [w432 w443]
          tunnel: [w435 0.0 ("Remaining Time")] -> w402
          tunnel: [w434 100.0] -> w408
          tunnel: [w431 w442] -> w406
          tunnel: [w430 w442] -> w405
          tunnel: ["Process Wait" "Process End"] -> w404
          frame False {
            n221 = Divide(x=w433, y=w432) -> (x/y=w438:dbl)
            n222 = Number To Decimal String(number=w433) -> (decimal integer string=w431:string)  [unwired: 1 in]
            n223 = Number To Decimal String(number=w432) -> (decimal integer string=w430:string)  [unwired: 1 in]
            n224 = Multiply(x=w438, y=100.0) -> (x*y=w434:dbl)
          }
          frame True {
            n225 = Number To Decimal String(number=w443) -> (decimal integer string=w442:string)  [unwired: 1 in]
          }
        }
        "Total Process" <- w405
        "Current Process" <- w406
        n226 = Wait (ms)(milliseconds to wait=u32 200) -> ()  [unwired: 1 out]
        n227 = Round Toward +Infinity(x=w402) -> (ceil(x): smallest int >= x=→"Remaining Time(s)":dbl)
        n228 = Increment(x=w408) -> (x+1=w421:dbl)
        n229 = Bundle(cluster=cluster{dbl, i32} {0.0, 7611776}, w408) -> (w420:cluster{dbl, i32})  [unwired: 1 in]
        n230 = Replace Array Subset(array=cluster{dbl, u32}[] [{0.0, 14869218}, {1.0, 7611776}, {100.0, 14869218}, {100.0, 14869218}] ("Scale.Marker Values[]"), new element=w420, index=1) -> (w422:cluster{dbl, u32}[])
        n231 = Bundle(cluster=cluster{dbl, i32} {0.0, 14869218}, w421) -> (w423:cluster{dbl, i32})  [unwired: 1 in]
        n232 = Replace Array Subset(array=w422, new element=w423, index=2) -> (w424:cluster{dbl, u32}[])
        n233 = property on="Gauge" class="Knob (strict)"("Scale.MarkerVals[]"=w424) -> ()  [unwired: 2 in, 2 out]
        n234 = call "Enqueue.vi"("Error In"=w413, "State"=w404, "Queue in"=w407) -> ("Error Out"=w412:errorcluster)  [unwired: 7 in, 1 out]
      }
      frame "Process End" {
        n235 = Generate User Event(user event=w447, event data cluster="Process End" ("event data"), error in=w449) -> (error out=w448:errorcluster)  [unwired: 1 in, 1 out]
        n236 = call "Process Msg"() -> ()  [unwired: 10 in, 2 out]
      }
      frame "------Function------" {
      }
      frame "BL2" {
        n237 = Variant To Data(error in=w457, type=FALSE, Variant=w456) -> (data=w452:bool, error out=w454:errorcluster)
        "BL2" <- w452
        n238 = call "BL2.vi"("Error In"=w454, "On/Off"=w452) -> ("Error Out"=w453:errorcluster)  [unwired: 9 in]
      }
      frame "BL1" {
        n239 = Variant To Data(error in=w464, type=FALSE, Variant=w463) -> (data=w459:bool, error out=w461:errorcluster)
        "BL1" <- w459
        n240 = call "BL1.vi"("Error In"=w461, "On/Off"=w459) -> ("Error Out"=w460:errorcluster)  [unwired: 9 in]
      }
      frame "BR1" {
        n241 = Variant To Data(error in=w471, type=FALSE, Variant=w470) -> (data=w466:bool, error out=w468:errorcluster)
        "BR1" <- w466
        n242 = call "BR1.vi"("Error In"=w468, "On/Off"=w466) -> ("Error Out"=w467:errorcluster)  [unwired: 9 in]
      }
      frame "BR2" {
        n243 = Variant To Data(error in=w478, type=FALSE, Variant=w477) -> (data=w473:bool, error out=w475:errorcluster)
        "BR2" <- w473
        n244 = call "BR2.vi"("Error In"=w475, "On/Off"=w473) -> ("Error Out"=w474:errorcluster)  [unwired: 9 in]
      }
      frame "V1+BR1" {
        n245 = Variant To Data(error in=w485, type=FALSE, Variant=w484) -> (data=w480:bool, error out=w482:errorcluster)
        "V1" <- w480
        n246 = local write "BR1"(w480) -> ()
        n247 = call "V1+BR1.vi"("Error In"=w482, "On/Off"=w480) -> ("Error Out"=w481:errorcluster)  [unwired: 9 in]
      }
      frame "V2+BR2" {
        n248 = Variant To Data(error in=w492, type=FALSE, Variant=w491) -> (data=w487:bool, error out=w489:errorcluster)
        "V2" <- w487
        n249 = local write "BR2"(w487) -> ()
        n250 = call "V2+BR2.vi"("Error In"=w489, "On/Off"=w487) -> ("Error Out"=w488:errorcluster)  [unwired: 9 in]
      }
      frame "REA" {
        n251 = Variant To Data(error in=w500, type=FALSE, Variant=w499) -> (data=w494:bool, error out=w497:errorcluster)
        "REA" <- w494
        n252 = call "REA.vi"("Error In"=w497, "On/Off"=w494) -> ("Error Out"=w496:errorcluster)  [unwired: 9 in]
        n253 = case shown="False" w494 {
          tunnel: w496 -> [w504 w507]
          tunnel: [w503 w506] -> w495
          frame True {
            n254 = call "Move.vi"("Error In"=w504, "Position"=T3."Position 2") -> ("Error Out"=w503:errorcluster)  [unwired: 9 in]
          }
          frame False {
            n255 = call "Move.vi"("Error In"=w507, "Position"=T3."Position 1") -> ("Error Out"=w506:errorcluster)  [unwired: 9 in]
          }
        }
      }
      frame "FW1/2" {
        n256 = Variant To Data(error in=w513, type=FALSE, Variant=w512) -> (data=w508:bool, error out=w510:errorcluster)
        "FW 1" <- w508
        "FW 2" <- w508
        n257 = call "FW12.vi"("Error In"=w510, "On/Off"=w508) -> ("Error Out"=w509:errorcluster)  [unwired: 9 in]
      }
      frame "SW1/2" {
        n258 = Variant To Data(error in=w520, type=FALSE, Variant=w519) -> (data=w515:bool, error out=w517:errorcluster)
        "SW 1" <- w515
        "SW 2" <- w515
        n259 = call "SW12.vi"("Error In"=w517, "On/Off"=w515) -> ("Error Out"=w516:errorcluster)  [unwired: 9 in]
      }
      frame "Buffer Load L" {
        n260 = call "Busy.vi"("Error In"=w523) -> ("Error Out"=w522:errorcluster)  [unwired: 10 in]
        n261 = call "Enqueue.vi"("Error In"=w522, "State"="Buffer Load L Wait", "Queue in"=w528) -> ("Error Out"=w529:errorcluster)  [unwired: 7 in, 1 out]
        n262 = call "Buffer Load L.vi"("Error In"=w529, "On/Off"=TRUE) -> ("Error Out"=w526:errorcluster)  [unwired: 9 in]
        n263 = Tick Count (ms)() -> (millisecond timer value=w524:u32)
        n264 = Bundle By Name(cluster=w531, "Tick Count"=w524) -> (w525:cluster{"Tick Count":u32})
      }
      frame "Buffer Load L Wait" {
        n265 = Unbundle By Name(w541) -> ("Tick Count"=w540:u32)
        n266 = Tick Count (ms)() -> (millisecond timer value=w539:u32)
        n267 = Subtract(x=w539, y=w540) -> (x-y=w538:u32)
        n268 = Greater Or Equal?(x=w538, y=u32 10000) -> (x >= y?=w536:bool)
        n269 = case shown="True" w536 {
          tunnel: w535 -> [w545 w549]
          tunnel: [w544 w546] -> w534
          tunnel: w533 -> [w543 _]
          frame False {
            n270 = call "Enqueue.vi"("Error In"=w545, "State"="Buffer Load L Wait", "Queue in"=w543) -> ("Error Out"=w544:errorcluster)  [unwired: 7 in, 1 out]
          }
          frame True {
            n271 = call "Display Message to User"() -> ()  [unwired: 10 in, 2 out]
            n272 = call "Buffer Load L.vi"("Error In"=w549, "On/Off"=FALSE) -> ("Error Out"=w547:errorcluster)  [unwired: 9 in]
            n273 = call "Unbusy.vi"("Error In"=w547) -> ("Error Out"=w546:errorcluster)  [unwired: 10 in]
          }
        }
        n274 = Wait (ms)(milliseconds to wait=u32 100) -> ()  [unwired: 1 out]
      }
      frame "Buffer Load R" {
        n275 = call "Busy.vi"("Error In"=w551) -> ("Error Out"=w550:errorcluster)  [unwired: 10 in]
        n276 = call "Enqueue.vi"("Error In"=w550, "State"="Buffer Load R Wait", "Queue in"=w558) -> ("Error Out"=w554:errorcluster)  [unwired: 7 in, 1 out]
        n277 = call "Buffer Load R.vi"("Error In"=w554, "On/Off"=TRUE) -> ("Error Out"=w553:errorcluster)  [unwired: 9 in]
        n278 = Tick Count (ms)() -> (millisecond timer value=w555:u32)
        n279 = Bundle By Name(cluster=w559, "Tick Count"=w555) -> (w556:cluster{"Tick Count":u32})
      }
      frame "Buffer Load R Wait" {
        n280 = Unbundle By Name(w569) -> ("Tick Count"=w568:u32)
        n281 = Tick Count (ms)() -> (millisecond timer value=w567:u32)
        n282 = Subtract(x=w567, y=w568) -> (x-y=w566:u32)
        n283 = Greater Or Equal?(x=w566, y=u32 10000) -> (x >= y?=w564:bool)
        n284 = case shown="True" w564 {
          tunnel: w563 -> [w573 w577]
          tunnel: [w572 w574] -> w562
          tunnel: w561 -> [w571 _]
          frame False {
            n285 = call "Enqueue.vi"("Error In"=w573, "State"="Buffer Load L Wait", "Queue in"=w571) -> ("Error Out"=w572:errorcluster)  [unwired: 7 in, 1 out]
          }
          frame True {
            n286 = call "Buffer Load R.vi"("Error In"=w577, "On/Off"=FALSE) -> ("Error Out"=w575:errorcluster)  [unwired: 9 in]
            n287 = call "Unbusy.vi"("Error In"=w575) -> ("Error Out"=w574:errorcluster)  [unwired: 10 in]
          }
        }
        n288 = Wait (ms)(milliseconds to wait=u32 100) -> ()  [unwired: 1 out]
      }
      frame "------Close------" {
      }
      frame "Close" {
        n289 = Release Queue(queue=w582, error in (no error)=w584) -> (error out=w583:errorcluster)  [unwired: 1 in, 2 out]
      }
    }
  }
  n290 = Merge Errors(w27, w26) -> (w24:errorcluster)
  n291 = Unregister For Events(event registration refnum=w25, error in=w24) -> (error out=w23:errorcluster)
  n292 = Destroy User Event(user event=w20, error in=w23) -> (error out=→"error out":errorcluster)
